vi "DB_Action-AddModule.vi"(8 "error in":errorcluster, 10 "UUT输入":T1) -> (0 "error out":errorcluster)   [LabVIEW 2015, in "Settings-Style.lvlib"]
uses:
  Settings-Style.lvlib
  1_Ctl/DB_UUT.ctl
  1_ctl/Ctl-Color.ctl
panel:
  out "Result":string caption="结果"
  # "Style Settings"
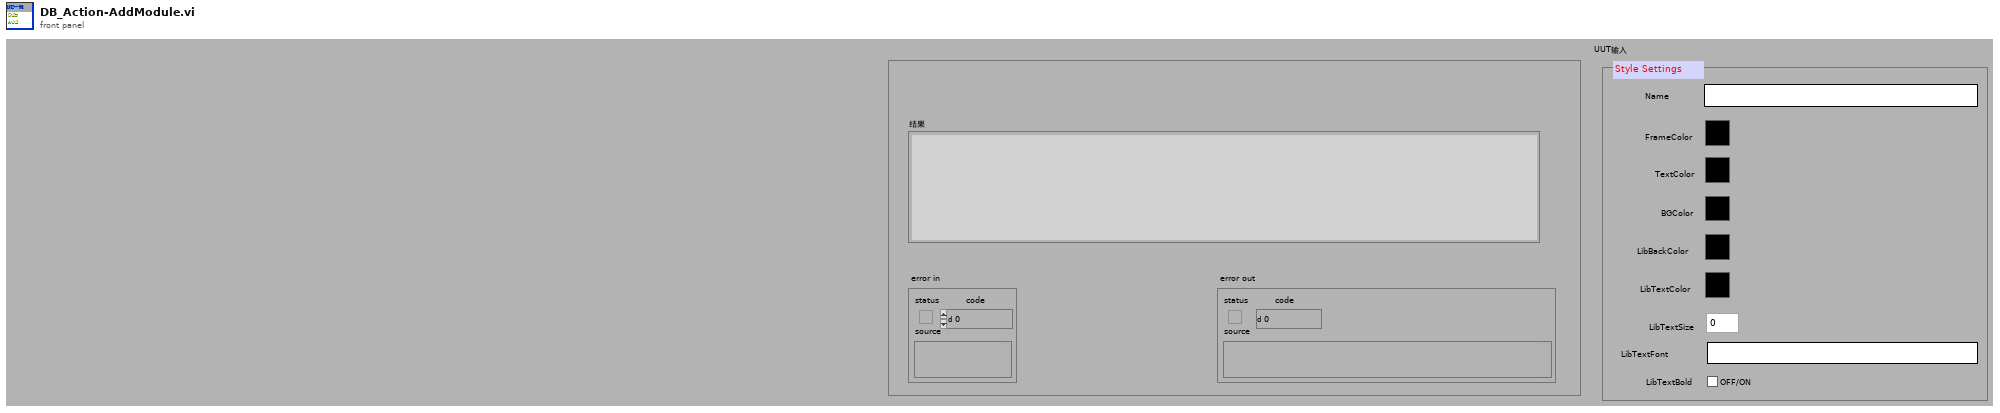
[diagram p1: front panel]
types:
  T1 = typedef "Settings-Style.lvlib/DB_UUT.ctl" = cluster{"Name":string, "FrameColor":T2, "TextColor":T2, "BGColor":T2, "LibBackColor":T2, "LibTextColor":T2, "LibTextSize":u32, "LibTextFont":string, "LibTextBold":bool}
  T2 = typedef "Ctl-Color.ctl" = u32
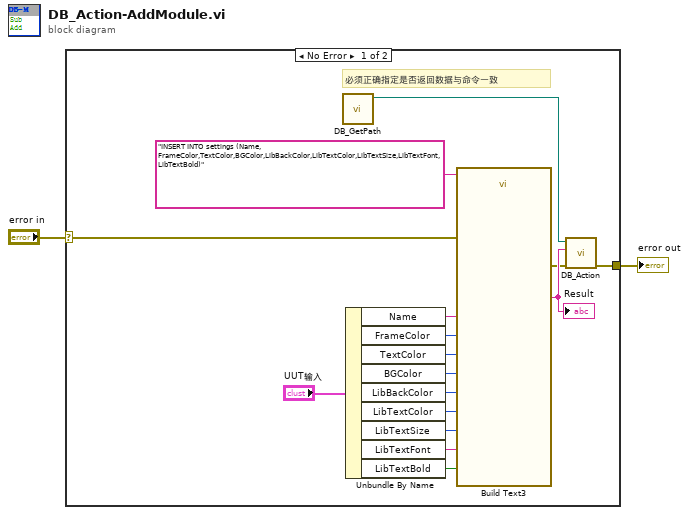
[diagram p0: block diagram]
diagram:
  n1 = case shown="No Error" "error in" {
    selector: "error in" -> [w3 w19]
    tunnel: [w18 w19] -> w2
    frame No Error {
      # "必须正确指定是否返回数据与命令一致"
      n2 = call "DB_GetPath.vi"() -> ("appended path"=w16:path)  [unwired: 11 in]
      n3 = Unbundle By Name("UUT输入") -> ("Name"=w6:string, "FrameColor"=w7:T2, "TextColor"=w8:T2, "BGColor"=w9:T2, "LibBackColor"=w10:T2, "LibTextColor"=w11:T2, "LibTextSize"=w12:u32, "LibTextFont"=w13:string, "LibTextBold"=w14:bool)
      n4 = call "Build Text3"("Beginning Text"="INSERT INTO settings (Name, FrameColor,TextColor,BGColor,LibBackColor,LibTextColor,LibTextSize,LibTextFont,LibTextBold)", "Name"=w6, "FrameColor"=w7, "TextColor"=w8, "BGColor"=w9, "LibBackColor"=w10, "LibTextColor"=w11, "error in (no error)"=w3, "LibTextSize"=w12, "LibTextFont"=w13, "LibTextBold"=w14) -> ("Result"=w5:string, "error out"=w4:errorcluster)  [unwired: 15 in]
      "Result" <- w5
      n5 = call "DB_Action.vi"("error in"=w4, "Command Text"=w5, "路径"=w16) -> ("error out"=w18:errorcluster)  [unwired: 7 in, 1 out]
    }
    frame Error {
    }
  }
  "error out" <- w2
